vi "SentinelController v33.vi"() -> ()   [LabVIEW 2011] (continued)
                                n808 = local read "Number of data log entries hid"() -> (w3611:u32)
                                n809 = Unbundle(w3615) -> (w3614:i32)  [unwired: 3 out]
                                n810 = Unbundle(w3623) -> (w3621:u32)  [unwired: 1 out]
                                n811 = Unbundle(w3613) -> (w3612:i32)  [unwired: 3 out]
                                n812 = Unbundle(w3622) -> (w3620:u32)  [unwired: 1 out]
                                n813 = Number To Decimal String(number=w3629) -> (decimal integer string=w3638:string)  [unwired: 1 in]
                                n814 = Number To Decimal String(number=w3614) -> (decimal integer string=w3640:string)  [unwired: 1 in]
                                n815 = Number To Decimal String(number=w3630) -> (decimal integer string=w3642:string)  [unwired: 1 in]
                                n816 = Number To Decimal String(number=w3621) -> (decimal integer string=w3644:string)  [unwired: 1 in]
                                n817 = Number To Decimal String(number=w3631) -> (decimal integer string=w3647:string)  [unwired: 1 in]
                                n818 = Number To Decimal String(number=w3612) -> (decimal integer string=w3649:string)  [unwired: 1 in]
                                n819 = Number To Decimal String(number=w3632) -> (decimal integer string=w3651:string)  [unwired: 1 in]
                                n820 = Number To Decimal String(number=w3620) -> (decimal integer string=w3653:string)  [unwired: 1 in]
                                n821 = local read "Data log path and filename"() -> (w3619:path)
                                n822 = Get Date/Time String(want seconds? (F)=TRUE) -> (date string=w3627:string, time string=w3628:string)  [unwired: 2 in]
                                n823 = Number To Decimal String(number=w3611) -> (decimal integer string=w3616:string)  [unwired: 1 in]
                                n824 = Concatenate Strings(w3616, w3617, w3627, "   " ("string"), w3628, w3617, "H1 Alarming, H2 Nominal", w3617, w3636, w3617, "H1 Low Yield Alarm Limit: ", w3638, ", H1 yield = ", w3640, w3617, "H1 Low UPH Alarm Limit: ", w3642, ", H1 UPH = ", w3644, w3617, w3645, w3617, "H2 Low Yield Warning Limit: ", w3647, ", H2 yield = ", w3649, w3617, "H2 Low UPH Warning Limit: ", w3651, ", H2 UPH = ", w3653, w3617, w3617) -> (w3625:string)
                                n825 = call "SentinelDatalog.vi"("operation (0:open)"=T9."open", "String"=w3625, "data log path"=w3619) -> ()  [unwired: 8 in, 1 out]
                                }
                                frame "H1AH2W" {
                                w3664 = "\r\n"
                                n826 = local read "H1 online"() -> (w3681:bool)
                                n827 = local read "H2 online"() -> (w3682:bool)
                                n828 = local read "H2 UPH warning limit hid"() -> (w3679:dbl)
                                n829 = local read "H2  low yield warning"() -> (w3678:dbl)
                                n830 = local read "H1 UPH alarm limit hid"() -> (w3677:dbl)
                                n831 = local read "H1 low yield alarm"() -> (w3676:dbl)
                                n832 = local read "H1 UPH"() -> (w3670:cluster{u32, u32})
                                n833 = local read "H2 UPH"() -> (w3669:cluster{u32, u32})
                                n834 = local read "YieldMon"() -> (w3662:cluster{i32, i32, i32, i32})
                                n835 = local read "YieldMon"() -> (w3660:cluster{i32, i32, i32, i32})
                                n836 = case shown="True" w3681 {
                                tunnel: ["H1 Off-Line" "H1 On-Line"] -> w3683
                                frame False {
                                }
                                frame True {
                                }
                                }
                                n837 = case shown="True" w3682 {
                                tunnel: ["H2 Off-Line" "H2 On-Line"] -> w3692
                                frame False {
                                }
                                frame True {
                                }
                                }
                                n838 = local read "Number of data log entries hid"() -> (w3658:u32)
                                n839 = Unbundle(w3662) -> (w3661:i32)  [unwired: 3 out]
                                n840 = Unbundle(w3670) -> (w3668:u32)  [unwired: 1 out]
                                n841 = Unbundle(w3660) -> (w3659:i32)  [unwired: 3 out]
                                n842 = Unbundle(w3669) -> (w3667:u32)  [unwired: 1 out]
                                n843 = Number To Decimal String(number=w3676) -> (decimal integer string=w3685:string)  [unwired: 1 in]
                                n844 = Number To Decimal String(number=w3661) -> (decimal integer string=w3687:string)  [unwired: 1 in]
                                n845 = Number To Decimal String(number=w3677) -> (decimal integer string=w3689:string)  [unwired: 1 in]
                                n846 = Number To Decimal String(number=w3668) -> (decimal integer string=w3691:string)  [unwired: 1 in]
                                n847 = Number To Decimal String(number=w3678) -> (decimal integer string=w3694:string)  [unwired: 1 in]
                                n848 = Number To Decimal String(number=w3659) -> (decimal integer string=w3696:string)  [unwired: 1 in]
                                n849 = Number To Decimal String(number=w3679) -> (decimal integer string=w3698:string)  [unwired: 1 in]
                                n850 = Number To Decimal String(number=w3667) -> (decimal integer string=w3700:string)  [unwired: 1 in]
                                n851 = local read "Data log path and filename"() -> (w3666:path)
                                n852 = Get Date/Time String(want seconds? (F)=TRUE) -> (date string=w3674:string, time string=w3675:string)  [unwired: 2 in]
                                n853 = Number To Decimal String(number=w3658) -> (decimal integer string=w3663:string)  [unwired: 1 in]
                                n854 = Concatenate Strings(w3663, w3664, w3674, "   " ("string"), w3675, w3664, "H1 Alarming, H2 Warning", w3664, w3683, w3664, "H1 Low Yield Alarm Limit: ", w3685, ", H1 yield = ", w3687, w3664, "H1 Low UPH Alarm Limit: ", w3689, ", H1 UPH = ", w3691, w3664, w3692, w3664, "H2 Low Yield Warning Limit: ", w3694, ", H2 yield = ", w3696, w3664, "H2 Low UPH Warning Limit: ", w3698, ", H2 UPH = ", w3700, w3664) -> (w3672:string)
                                n855 = call "SentinelDatalog.vi"("operation (0:open)"=T9."open", "String"=w3672, "data log path"=w3666) -> ()  [unwired: 8 in, 1 out]
                                }
                                frame "H1AH2A" {
                                w3711 = "\r\n"
                                n856 = local read "H1 online"() -> (w3728:bool)
                                n857 = local read "H2 online"() -> (w3729:bool)
                                n858 = local read "H1 UPH alarm limit hid"() -> (w3724:dbl)
                                n859 = local read "H2 UPH alarm limit hid"() -> (w3726:dbl)
                                n860 = local read "H1 low yield alarm"() -> (w3723:dbl)
                                n861 = local read "H1 UPH"() -> (w3717:cluster{u32, u32})
                                n862 = local read "H2 low yield alarm"() -> (w3725:dbl)
                                n863 = local read "H2 UPH"() -> (w3716:cluster{u32, u32})
                                n864 = local read "YieldMon"() -> (w3709:cluster{i32, i32, i32, i32})
                                n865 = local read "YieldMon"() -> (w3708:cluster{i32, i32, i32, i32})
                                n866 = case shown="True" w3728 {
                                tunnel: ["H1 Off-Line" "H1 On-Line"] -> w3730
                                frame False {
                                }
                                frame True {
                                }
                                }
                                n867 = case shown="True" w3729 {
                                tunnel: ["H2 Off-Line" "H2 On-Line"] -> w3739
                                frame False {
                                }
                                frame True {
                                }
                                }
                                n868 = local read "Number of data log entries hid"() -> (w3705:u32)
                                n869 = Unbundle(w3709) -> (w3706:i32)  [unwired: 3 out]
                                n870 = Unbundle(w3717) -> (w3715:u32)  [unwired: 1 out]
                                n871 = Unbundle(w3708) -> (w3707:i32)  [unwired: 3 out]
                                n872 = Unbundle(w3716) -> (w3714:u32)  [unwired: 1 out]
                                n873 = Number To Decimal String(number=w3723) -> (decimal integer string=w3732:string)  [unwired: 1 in]
                                n874 = Number To Decimal String(number=w3706) -> (decimal integer string=w3734:string)  [unwired: 1 in]
                                n875 = Number To Decimal String(number=w3724) -> (decimal integer string=w3736:string)  [unwired: 1 in]
                                n876 = Number To Decimal String(number=w3715) -> (decimal integer string=w3738:string)  [unwired: 1 in]
                                n877 = Number To Decimal String(number=w3725) -> (decimal integer string=w3741:string)  [unwired: 1 in]
                                n878 = Number To Decimal String(number=w3707) -> (decimal integer string=w3743:string)  [unwired: 1 in]
                                n879 = Number To Decimal String(number=w3726) -> (decimal integer string=w3745:string)  [unwired: 1 in]
                                n880 = Number To Decimal String(number=w3714) -> (decimal integer string=w3747:string)  [unwired: 1 in]
                                n881 = local read "Data log path and filename"() -> (w3713:path)
                                n882 = Get Date/Time String(want seconds? (F)=TRUE) -> (date string=w3721:string, time string=w3722:string)  [unwired: 2 in]
                                n883 = Number To Decimal String(number=w3705) -> (decimal integer string=w3710:string)  [unwired: 1 in]
                                n884 = Concatenate Strings(w3710, w3711, w3721, "   " ("string"), w3722, w3711, "H1 Alarming, H2 Alarming", w3711, w3730, w3711, "H1 Low Yield Alarm Limit: ", w3732, ", H1 yield = ", w3734, w3711, "H1 Low UPH Alarm Limit: ", w3736, ", H1 UPH = ", w3738, w3711, w3739, w3711, "H2 Low Yield Alarm Limit: ", w3741, ", H2 yield = ", w3743, w3711, "H2 Low UPH Alarm Limit: ", w3745, ", H2 UPH = ", w3747, w3711, w3711) -> (w3719:string)
                                n885 = call "SentinelDatalog.vi"("operation (0:open)"=T9."open", "String"=w3719, "data log path"=w3713) -> ()  [unwired: 8 in, 1 out]
                                }
                                }
                                }
                                frame #2 {
                                n886 = Wait (ms)(milliseconds to wait=u32 100) -> ()  [unwired: 1 out]
                                }
                                frame #3 {
                                n887 = local read "Enable electronic notification of alarms"() -> (w3753:bool)
                                n888 = case shown="True" w3753 {
                                frame False {
                                }
                                frame True {
                                n889 = stacked-sequence {
                                frame #0 {
                                # "Email"
                                n890 = local read "Enable email notification"() -> (w3756:bool)
                                n891 = local read "Number of email alerts"() -> (w3755:u32)
                                n892 = Increment(x=w3755) -> (x+1=w3754:u32)
                                n893 = local write "Number of email alerts"(w3754) -> ()
                                n894 = case shown="True" w3756 {
                                frame False {
                                }
                                frame True {
                                n895 = flat-sequence {
                                tunnel: [w3763] -> w3758
                                tunnel: [w3771] -> w3757
                                tunnel: w3758 -> [w3771]
                                tunnel: w3757 -> [w3772]
                                frame #0 {
                                n896 = local read "Data log path and filename"() -> (w3768:path)
                                n897 = local read "Number of email alerts"() -> (w3762:u32)
                                n898 = Number To Decimal String(number=w3762) -> (decimal integer string=w3761:string)  [unwired: 1 in]
                                n899 = Strip Path(path=w3768) -> (stripped path=w3766:path, name=w3760:string)
                                n900 = Path To String(path=w3766) -> (string=w3765:string)
                                n901 = Concatenate Strings(w3765, "\\sent_#" ("string"), w3761, "_" ("string"), w3760) -> (w3769:string)
                                n902 = String To Path(string=w3769) -> (path=w3764:path)
                                n903 = Copy(10:w3764, 11:w3768) -> (3:w3763:path)  [unwired: 3 in, 2 out]
                                }
                                frame #1 {
                                n904 = Wait (ms)(milliseconds to wait=u32 1000) -> ()  [unwired: 1 out]
                                }
                                frame #2 {
                                n905 = local read "Email alert - engineer"() -> (w3774:string)
                                n906 = local read "Email alert - CC"() -> (w3773:string)
                                n907 = local read "Email alert - message"() -> (w3775:string)
                                n908 = call "email_alert.vi"("Email Alert - Message"=w3775, "Email Alert - Engineer"=w3774, "Email Alert - CC"=w3773, "Email ALert - Attachment"=w3772) -> ()  [unwired: 8 in]
                                }
                                }
                                }
                                }
                                }
                                frame #1 {
                                n909 = Wait (ms)(milliseconds to wait=u32 200) -> ()  [unwired: 1 out]
                                }
                                frame #2 {
                                # "text"
                                n910 = local read "Enable text notification"() -> (w3777:bool)
                                n911 = case shown="True" w3777 {
                                frame False {
                                }
                                frame True {
                                n912 = local read "Number of text alerts"() -> (w3781:u32)
                                n913 = Increment(x=w3781) -> (x+1=w3780:u32)
                                n914 = local write "Number of text alerts"(w3780) -> ()
                                n915 = local read "Number of email alerts"() -> (w3790:u32)
                                n916 = local read "Carrier"() -> (w3783:enum16{"T-Mobile", "AT&T", "Verizon", "Sprint"})
                                n917 = local read "Phone number"() -> (w3782:string)
                                n918 = local read "Body"() -> (w3779:string)
                                n919 = local read "Lot number"() -> (w3784:string)
                                n920 = local read "Subject"() -> (w3778:string)
                                n921 = Number To Decimal String(number=w3790) -> (decimal integer string=w3786:string)  [unwired: 1 in]
                                n922 = Concatenate Strings(w3779, ", # " ("string"), w3786, ", Lot Number: " ("string"), w3784) -> (w3791:string)
                                n923 = local write "Notifications Lot Display"(w3784) -> ()
                                n924 = call <userlib>:"Send SMS 2009.vi"("Body"=w3791, "Carrier"=w3783, "Subject"=w3778, "phone number"=w3782, "smtp server"="smtp.gmail.com", "password"="sentinelcontroller", "email username"="sentinelcontroller@gmail.com") -> ("Error Out"=w3789:errorcluster)  [unwired: 4 in]
                                n925 = Unbundle By Name(w3789) -> ("status"=w3788:bool)
                                n926 = case shown="True" w3788 {
                                frame False {
                                }
                                frame True {
                                n927 = One Button Dialog(message="Warning:\nError sending text message!\nTry changing the settings or\nswitch to email method", button name ("OK")="Dismiss") -> ()  [unwired: 1 out]
                                }
                                }
                                }
                                }
                                }
                                }
                                }
                                }
                                }
                                frame #4 {
                                n928 = Wait (ms)(milliseconds to wait=u32 100) -> ()  [unwired: 1 out]
                                }
                              }
                            }
                          }
                        }
                      }
                    }
                  }
                }
              }
              n929 = Wait (ms)(milliseconds to wait=u32 100) -> ()  [unwired: 1 out]
            }
            n930 = local read "Yield averaging"() -> (w350:u32)
            n931 = local read "UPH averaging"() -> (w349:u32)
            n932 = local read "Yield averaging"() -> (w351:u32)
            n933 = local read "UPH averaging"() -> (w352:u32)
            n934 = Initialize Array(w347, w350) -> (w348:i32[])
            n935 = Initialize Array(w346, w349) -> (w345:dbl[])
            n936 = Initialize Array(w354, w351) -> (w353:i32[])
            n937 = Initialize Array(w355, w352) -> (w356:dbl[])
            n938 = while {
              shift-right: [w3060] -> _
              shift-left: w346 -> [w3066]
              shift-right: [w3061] -> _
              shift-left: w345 -> [w3065]
              shift-right: [w3062] -> _
              shift-left: w347 -> [w3059]
              shift-right: [w3063] -> _
              shift-left: w348 -> [w3064]
              stop <- w3057 stop-if-true
              # "if there is now a lock, it is unlikely that the test time is going to be less than 100ms,\nso this is a relatively slow loop"
              n939 = local read "H2 Lock"() -> (w3056:bool)
              n940 = Wait (ms)(milliseconds to wait=u32 50) -> ()  [unwired: 1 out]
              n941 = case shown="True" w3056 {
                tunnel: w3066 -> [w3071 w3096]
                tunnel: w3065 -> [w3070 w3091]
                tunnel: w3064 -> [w3068 w3088]
                tunnel: [w3068 w3082] -> w3063
                tunnel: [w3069 w3080] -> w3062
                tunnel: [w3070 w3079] -> w3061
                tunnel: [w3071 w3078] -> w3060
                tunnel: w3059 -> [w3069 w3077]
                frame False {
                  n942 = local write "Calc H1 UPH"(u32 0 ("Sim H1 UPH")) -> ()
                }
                frame True {
                  n943 = flat-sequence {
                    tunnel: w3088 -> [w3099]
                    tunnel: w3077 -> [w3100]
                    tunnel: w3091 -> [w3101]
                    tunnel: w3096 -> [w3102]
                    tunnel: [w3102] -> w3087
                    tunnel: [w3101] -> w3086
                    tunnel: [w3100] -> w3085
                    tunnel: [w3099] -> w3084
                    tunnel: [w3115] -> w3095
                    tunnel: [w3114] -> w3092
                    tunnel: [w3113] -> w3090
                    tunnel: [w3112] -> w3089
                    tunnel: w3087 -> [w3115]
                    tunnel: w3086 -> [w3114]
                    tunnel: w3085 -> [w3113]
                    tunnel: w3084 -> [w3112]
                    tunnel: w3095 -> [w3141]
                    tunnel: [w3141] -> w3094
                    tunnel: [w3140] -> w3093
                    tunnel: w3092 -> [w3140]
                    tunnel: w3090 -> [w3130]
                    tunnel: w3089 -> [w3129]
                    tunnel: [w3128] -> w3083
                    tunnel: [w3127] -> w3081
                    tunnel: w3094 -> [w3167]
                    tunnel: w3093 -> [w3168]
                    tunnel: w3083 -> [w3186]
                    tunnel: w3081 -> [w3185]
                    tunnel: [w3186] -> w3076
                    tunnel: [w3185] -> w3075
                    tunnel: [w3164] -> w3074
                    tunnel: [w3163] -> w3073
                    tunnel: [w3201] -> w3078
                    tunnel: [w3202] -> w3079
                    tunnel: [w3203] -> w3080
                    tunnel: [w3204] -> w3082
                    tunnel: w3076 -> [w3204]
                    tunnel: w3075 -> [w3203]
                    tunnel: w3074 -> [w3202]
                    tunnel: w3073 -> [w3201]
                    frame #0 {
                      n944 = local read "H2 loop counter hid"() -> (w3097:u32)
                      n945 = Equal To 0?(x=w3097) -> (x = 0?=w3098:bool)
                      n946 = case shown="True" w3098 {
                        frame False {
                        }
                        frame True {
                          # "H2 first pass init"
                          n947 = local write "H2 Device Count"(0.0 ("H2 Device Count")) -> ()
                          n948 = local write "H2 measured  Index Time"(0.0 ("H2 Index Time")) -> ()
                          n949 = local write "H2 measured Test Time"(0.0 ("H2 Test Time")) -> ()
                          n950 = local write "H2 measured Wait Time"(0.0 ("H2 Wait Time")) -> ()
                          n951 = local read "H2 low UPH alarm (%)"() -> (w3106:dbl)
                          n952 = Divide(x=w3106, y=100.0) -> (x/y=w3105:dbl)
                          n953 = Bundle(0.0, w3105) -> (w3103:cluster{dbl, dbl})  [unwired: 1 in]
                          n954 = local write "H2 UPH"(w3103) -> ()
                        }
                      }
                    }
                    frame #1 {
                      # "H2 testing"
                      n955 = while {
                        stop <- w3119 stop-if-true
                        n956 = local read "H2 Lock"() -> (w3123:bool)
                        n957 = local read "POWER"() -> (w3118:bool)
                        n958 = local read "Run"() -> (w3116:bool)
                        n959 = Not(x=w3123) -> (.not. x?=w3117:bool)
                        n960 = Not(x=w3118) -> (.not. x?=w3121:bool)
                        n961 = Not(x=w3116) -> (.not. x?=w3120:bool)
                        n962 = Compound Arithmetic op=OR(w3117, w3121, w3120) -> (w3119:bool)
                        n963 = Wait (ms)(milliseconds to wait=u32 1) -> ()  [unwired: 1 out]
                      }
                    }
                    frame #2 {
                      n964 = local read "H2 cycle yield hid"() -> (w3124:dbl)
                      n965 = local read "H2 loop counter hid"() -> (w3125:u32)
                      n966 = local read "Yield averaging"() -> (w3126:u32)
                      n967 = local read "H2 low yield alarm"() -> (w3139:dbl)
                      n968 = local read "YieldMon"() -> (w3132:cluster{i32, i32, i32, i32})
                      n969 = local read "H2  low yield warning"() -> (w3138:dbl)
                      n970 = call "moving_avg_core.vi"("Array in"=w3129, "avg"=w3126, "accumulator in"=w3130, "i"=w3125, "data in"=w3124) -> ("Array out"=w3128:dbl[], "accumulator out"=w3127:dbl, "rolling avg out"=w3133:dbl)  [unwired: 4 in]
                      n971 = Unbundle(w3132) -> (w3131:i32)  [unwired: 3 out]
                      n972 = Less?(x=w3133, y=w3138) -> (x < y?=w3137:bool)
                      n973 = case shown="True" w3137 {
                        tunnel: w3133 -> [_ w3146]
                        tunnel: w3139 -> [_ w3145]
                        frame False {
                          n974 = local write "H2 nominal"(TRUE ("H1 nominal")) -> ()
                          n975 = local write "H2 warning"(FALSE ("H1 warning")) -> ()
                          n976 = local write "H2 alarm"(FALSE ("H1 warning")) -> ()
                        }
                        frame True {
                          n977 = Less?(x=w3146, y=w3145) -> (x < y?=w3147:bool)
                          n978 = case shown="True" w3147 {
                            frame False {
                              n979 = local write "H2 nominal"(FALSE ("H1 nominal")) -> ()
                              n980 = local write "H2 warning"(TRUE ("H1 warning")) -> ()
                              n981 = local write "H2 alarm"(FALSE ("H1 warning")) -> ()
                            }
                            frame True {
                              n982 = local read "H2 enable halt\non yield alarm"() -> (w3151:bool)
                              n983 = local write "H2 nominal"(FALSE ("H1 nominal")) -> ()
                              n984 = local write "H2 alarm"(TRUE ("H1 warning")) -> ()
                              n985 = local write "H2 warning"(FALSE ("H1 warning")) -> ()
                              n986 = case shown="True" w3151 {
                                frame False {
                                }
                                frame True {
                                n987 = local write "H2 online"(FALSE ("H1 Online")) -> ()
                                }
                              }
                            }
                          }
                        }
                      }
                      n988 = local read "H1 low yield alarm"() -> (w3136:dbl)
                      n989 = local read "H2 low yield alarm"() -> (w3135:dbl)
                      n990 = Bundle(w3131, "rolling avg out"=w3133, "H1 low yield alarm"=w3136, "H2 low yield alarm"=w3135) -> (w3134:T11)  [unwired: 1 in]
                      n991 = local write "YieldMon"(w3134) -> ()
                    }
                    frame #3 {
                      n992 = local read "H2 measured  Index Time"() -> (w3157:dbl)
                      n993 = local read "H2 measured Wait Time"() -> (w3156:dbl)
                      n994 = local read "H2 measured Test Time"() -> (w3158:dbl)
                      n995 = local read "H2 parallelism"() -> (w3170:u32)
                      n996 = local read "H2 lot yield mon"() -> (w3184:dbl)
                      n997 = local write "H2 IT (scycle)"(w3157) -> ()
                      n998 = local write "H2 TT (s/cycle)"(w3158) -> ()
                      n999 = local write "H2 WT (s/cycle)"(w3156) -> ()
                      n1000 = Compound Arithmetic op=ADD(w3157, w3158, w3156) -> (w3173:dbl)
                      n1001 = Compound Arithmetic op=ADD(w3157, w3158) -> (w3169:dbl)
                      n1002 = Multiply(x=w3170, y=3600.0 ("x")) -> (x*y=w3172:dbl)
                      n1003 = Divide(x=w3172, y=w3173) -> (x/y=w3183:dbl)
                      n1004 = Divide(x=w3184, y=w3169) -> (x/y=w3162:dbl)
                      n1005 = local write "H2 Single Handler UPH hid"(w3162) -> ()
                      n1006 = local read "H2 low UPH warning (%)"() -> (w3180:dbl)
                      n1007 = local read "H2 loop counter hid"() -> (w3166:u32)
                      n1008 = local read "Yield averaging"() -> (w3165:u32)
                      n1009 = local read "H2 low UPH alarm (%)"() -> (w3175:dbl)
                      n1010 = property on="H2 UPH" class="Knob (strict)"() -> ("Scale.Maximum"=w3181:dbl)  [unwired: 2 in, 2 out]
                      n1011 = Divide(x=w3180, y=100.0) -> (x/y=w3179:dbl)
                      n1012 = call "moving_avg_core.vi"("Array in"=w3168, "avg"=w3165, "accumulator in"=w3167, "i"=w3166, "data in"=w3183) -> ("Array out"=w3164:dbl[], "accumulator out"=w3163:dbl, "rolling avg out"=w3182:dbl)  [unwired: 4 in]
                      n1013 = Multiply(x=w3181, y=w3179) -> (x*y=w3161:dbl)
                      n1014 = Divide(x=w3175, y=100.0) -> (x/y=w3177:dbl)
                      n1015 = local write "H2 UPH warning limit hid"(w3161) -> ()
                      n1016 = Less?(x=w3182, y=w3161) -> (x < y?=w3174:bool)
                      n1017 = Multiply(x=w3181, y=w3177) -> (x*y=w3160:dbl)
                      n1018 = case shown="True" w3174 {
                        tunnel: w3182 -> [_ w3191]
                        tunnel: w3160 -> [_ w3190]
                        frame False {
                          n1019 = local write "H2 nominal 2"(TRUE ("H1 nominal")) -> ()
                          n1020 = local write "H2 warning 2"(FALSE ("H1 warning")) -> ()
                          n1021 = local write "H2 alarm 2"(FALSE ("H1 warning")) -> ()
                        }
                        frame True {
                          n1022 = Less?(x=w3191, y=w3190) -> (x < y?=w3192:bool)
                          n1023 = case shown="True" w3192 {
                            frame False {
                              n1024 = local write "H2 nominal 2"(FALSE ("H1 nominal")) -> ()
                              n1025 = local write "H2 warning 2"(TRUE ("H1 warning")) -> ()
                              n1026 = local write "H2 alarm 2"(FALSE ("H1 warning")) -> ()
                            }
                            frame True {
                              n1027 = local read "H2 enable halt\non UPH alarm"() -> (w3196:bool)
                              n1028 = local write "H2 alarm 2"(TRUE ("H1 warning")) -> ()
                              n1029 = local write "H2 warning 2"(FALSE ("H1 warning")) -> ()
                              n1030 = local write "H2 nominal 2"(FALSE ("H1 nominal")) -> ()
                              n1031 = case shown="True" w3196 {
                                frame False {
                                }
                                frame True {
                                n1032 = local write "H2 online"(FALSE ("H1 Online")) -> ()
                                }
                              }
                            }
                          }
                        }
                      }
                      n1033 = local write "H2 UPH alarm limit hid"(w3160) -> ()
                      n1034 = Bundle("rolling avg out"=w3182, w3160) -> (w3159:cluster{"rolling avg out":dbl, dbl})  [unwired: 1 in]
                      n1035 = local write "H2 UPH"(w3159) -> ()
                    }
                    frame #4 {
                      n1036 = while {
                        stop <- w3206 continue-if-true
                        n1037 = local read "H2 Lock"() -> (w3206:bool)
                        n1038 = Wait (ms)(milliseconds to wait=u32 10) -> ()  [unwired: 1 out]
                      }
                    }
                  }
                }
              }
              n1039 = local read "POWER"() -> (w3058:bool)
              n1040 = Not(x=w3058) -> (.not. x?=w3057:bool)
            }
            n1041 = while {
              shift-right: [w3937] -> _
              shift-left: w355 -> [w3940]
              shift-right: [w3938] -> _
              shift-left: w356 -> [w3939]
              shift-right: [w3933] -> _
              shift-left: w354 -> [w3936]
              shift-right: [w3934] -> _
              shift-left: w353 -> [w3935]
              stop <- w3932 stop-if-true
              # "if there is now a lock, it is unlikely that the test time is going to be less than 100ms,\nso this is a relatively slow loop"
              n1042 = local read "H1 Lock"() -> (w3931:bool)
              n1043 = case shown="True" w3931 {
                tunnel: w3940 -> [w3946 w3971]
                tunnel: w3939 -> [w3945 w3966]
                tunnel: [w3945 w3965] -> w3938
                tunnel: [w3946 w3964] -> w3937
                tunnel: w3936 -> [w3944 w3962]
                tunnel: w3935 -> [w3943 w3960]
                tunnel: [w3943 w3958] -> w3934
                tunnel: [w3944 w3956] -> w3933
                frame False {
                  n1044 = local write "Calc H1 UPH"(u32 0 ("Sim H1 UPH")) -> ()
                }
                frame True {
                  n1045 = flat-sequence {
                    tunnel: w3960 -> [w3974]
                    tunnel: w3962 -> [w3975]
                    tunnel: w3966 -> [w3976]
                    tunnel: w3971 -> [w3977]
                    tunnel: [w3977] -> w3955
                    tunnel: [w3976] -> w3954
                    tunnel: [w3975] -> w3953
                    tunnel: [w3974] -> w3952
                    tunnel: [w3990] -> w3970
                    tunnel: [w3989] -> w3967
                    tunnel: [w3988] -> w3963
                    tunnel: [w3987] -> w3961
                    tunnel: w3955 -> [w3990]
                    tunnel: w3954 -> [w3989]
                    tunnel: w3953 -> [w3988]
                    tunnel: w3952 -> [w3987]
                    tunnel: w3970 -> [w4005]
                    tunnel: [w4005] -> w3969
                    tunnel: [w4004] -> w3968
                    tunnel: w3967 -> [w4004]
                    tunnel: w3963 -> [w4003]
                    tunnel: w3961 -> [w4002]
                    tunnel: [w4001] -> w3959
                    tunnel: [w4000] -> w3957
                    tunnel: w3969 -> [w4043]
                    tunnel: w3968 -> [w4042]
                    tunnel: w3959 -> [w4039]
                    tunnel: w3957 -> [w4038]
                    tunnel: [w4041] -> w3951
                    tunnel: [w4040] -> w3950
                    tunnel: [w4039] -> w3949
                    tunnel: [w4038] -> w3948
                    tunnel: [w4078] -> w3956
                    tunnel: [w4079] -> w3958
                    tunnel: [w4080] -> w3964
                    tunnel: [w4081] -> w3965
                    tunnel: w3951 -> [w4081]
                    tunnel: w3950 -> [w4080]
                    tunnel: w3949 -> [w4079]
                    tunnel: w3948 -> [w4078]
                    frame #0 {
                      n1046 = local read "H1 loop counter hid"() -> (w3973:u32)
                      n1047 = Equal To 0?(x=w3973) -> (x = 0?=w3972:bool)
                      n1048 = case shown="True" w3972 {
                        frame False {
                        }
                        frame True {
                          n1049 = local read "H1 low UPH alarm (%)"() -> (w3982:dbl)
                          n1050 = local write "H1 measured Index Time"(0.0 ("H1 Index Time")) -> ()
                          n1051 = local write "H1 measured Wait Time"(0.0 ("H1 Wait Time")) -> ()
                          n1052 = local write "H1 Device Count"(0.0 ("H1 Device Count")) -> ()
                          n1053 = local write "H1 measured Test Time"(0.0 ("H1 Test Time")) -> ()
                          n1054 = Divide(x=w3982, y=100.0) -> (x/y=w3980:dbl)
                          n1055 = Bundle("y"=0.0, w3980) -> (w3978:cluster{"y":dbl, dbl})  [unwired: 1 in]
                          n1056 = local write "H1 UPH"(w3978) -> ()
                        }
                      }
                    }
                    frame #1 {
                      # "H1 testing"
                      n1057 = while {
                        stop <- w3994 stop-if-true
                        n1058 = local read "H1 Lock"() -> (w3998:bool)
                        n1059 = local read "POWER"() -> (w3992:bool)
                        n1060 = local read "Run"() -> (w3991:bool)
                        n1061 = Wait (ms)(milliseconds to wait=u32 1) -> ()  [unwired: 1 out]
                        n1062 = Not(x=w3998) -> (.not. x?=w3993:bool)
                        n1063 = Not(x=w3992) -> (.not. x?=w3996:bool)
                        n1064 = Not(x=w3991) -> (.not. x?=w3995:bool)
                        n1065 = Compound Arithmetic op=OR(w3993, w3996, w3995) -> (w3994:bool)
                      }
                    }
                    frame #2 {
                      n1066 = local read "H1 cycle yield hid"() -> (w4008:dbl)
                      n1067 = local read "H1 loop counter hid"() -> (w4007:u32)
                      n1068 = local read "Yield averaging"() -> (w4006:u32)
                      n1069 = local read "H1 low yield warning"() -> (w4016:dbl)
                      n1070 = local read "H1 low yield alarm"() -> (w4014:dbl)
                      n1071 = call "moving_avg_core.vi"("Array in"=w4002, "avg"=w4006, "accumulator in"=w4003, "i"=w4007, "data in"=w4008) -> ("Array out"=w4001:dbl[], "accumulator out"=w4000:dbl, "rolling avg out"=w4011:dbl)  [unwired: 4 in]
                      n1072 = Less?(x=w4011, y=w4016) -> (x < y?=w4015:bool)
                      n1073 = case shown="True" w4015 {
                        tunnel: w4011 -> [_ w4022]
                        tunnel: w4014 -> [_ w4021]
                        frame False {
                          n1074 = local write "H1 alarm"(FALSE ("H1 warning")) -> ()
                          n1075 = local write "H1 warning"(FALSE ("H1 warning")) -> ()
                          n1076 = local write "H1 nominal"(TRUE ("H1 nominal")) -> ()
                        }
                        frame True {
                          n1077 = Less?(x=w4022, y=w4021) -> (x < y?=w4020:bool)
                          n1078 = case shown="True" w4020 {
                            frame False {
                              n1079 = local write "H1 alarm"(FALSE ("H1 warning")) -> ()
                              n1080 = local write "H1 warning"(TRUE ("H1 warning")) -> ()
                              n1081 = local write "H1 nominal"(FALSE ("H1 nominal")) -> ()
                            }
                            frame True {
                              n1082 = local read "H1 enable halt\non yield alarm"() -> (w4026:bool)
                              n1083 = local write "H1 nominal"(FALSE ("H1 nominal")) -> ()
                              n1084 = local write "H1 warning"(FALSE ("H1 warning")) -> ()
                              n1085 = local write "H1 alarm"(TRUE ("H1 warning")) -> ()
                              n1086 = case shown="True" w4026 {
                                frame False {
                                }
                                frame True {
                                n1087 = local write "H1 online"(FALSE ("H1 Online")) -> ()
                                }
                              }
                            }
                          }
                        }
                      }
                      n1088 = local read "YieldMon"() -> (w4010:cluster{i32, i32, i32, i32})
                      n1089 = local read "H1 low yield alarm"() -> (w4013:dbl)
                      n1090 = local read "H2 low yield alarm"() -> (w4012:dbl)
                      n1091 = Unbundle(w4010) -> (w3999:i32)  [unwired: 3 out]
                      n1092 = Bundle("rolling avg out"=w4011, w3999, "H1 low yield alarm"=w4013, "H2 low yield alarm"=w4012) -> (w4009:T12)  [unwired: 1 in]
                      n1093 = local write "YieldMon"(w4009) -> ()
                    }
                    frame #3 {
                      n1094 = local read "H1 measured Index Time"() -> (w4033:dbl)
                      n1095 = local read "H1 measured Wait Time"() -> (w4031:dbl)
                      n1096 = local read "H1 measured Test Time"() -> (w4032:dbl)
                      n1097 = local read "H1 parallelism"() -> (w4050:u32)
                      n1098 = local read "H1 loop counter hid"() -> (w4045:u32)
                      n1099 = local read "UPH averaging"() -> (w4044:u32)
                      n1100 = local read "H1 low UPH warning (%)"() -> (w4054:dbl)
                      n1101 = local write "H1 IT (s/cycle)"(w4033) -> ()
                      n1102 = local write "H1 TT (s/cycle)"(w4032) -> ()
                      n1103 = local write "H1 WT (s/cycle)"(w4031) -> ()
                      n1104 = Compound Arithmetic op=ADD(w4033, w4032, w4031) -> (w4046:dbl)
                      n1105 = Compound Arithmetic op=ADD(w4033, w4032) -> (w4053:dbl)
                      n1106 = Multiply(x=w4050, y=u32 3600 ("x")) -> (x*y=w4052:u32)
                      n1107 = Divide(x=w4052, y=w4053) -> (x/y=w4036:dbl)
                      n1108 = local read "H1 low UPH alarm (%)"() -> (w4059:dbl)
                      n1109 = local write "H1 Single Handler UPH hid"(w4036) -> ()
                      n1110 = property on="H1 UPH" class="Knob (strict)"() -> ("Scale.Maximum"=w4061:dbl)  [unwired: 2 in, 2 out]
                      n1111 = Divide(x=w4054, y=100.0) -> (x/y=w4055:dbl)
                      n1112 = Multiply(x=w4061, y=w4055) -> (x*y=w4034:dbl)
                      n1113 = Divide(x=w4059, y=100.0) -> (x/y=w4057:dbl)
                      n1114 = local write "H1 UPH warning limit hid"(w4034) -> ()
                      n1115 = Multiply(x=w4061, y=w4057) -> (x*y=w4035:dbl)
                      n1116 = local write "H1 UPH alarm limit hid"(w4035) -> ()
                      n1117 = local read "H1 parallelism"() -> (w4049:u32)
                      n1118 = Multiply(x=w4049, y=u32 3600 ("x")) -> (x*y=w4047:u32)
                      n1119 = Divide(x=w4047, y=w4046) -> (x/y=w4063:dbl)
                      n1120 = call "moving_avg_core.vi"("Array in"=w4042, "avg"=w4044, "accumulator in"=w4043, "i"=w4045, "data in"=w4063) -> ("Array out"=w4041:dbl[], "accumulator out"=w4040:dbl, "rolling avg out"=w4062:dbl)  [unwired: 4 in]
                      n1121 = Less?(x=w4062, y=w4034) -> (x < y?=w4060:bool)
                      n1122 = case shown="True" w4060 {
                        tunnel: w4062 -> [_ w4068]
                        tunnel: w4035 -> [_ w4067]
                        frame False {
                          n1123 = local write "H1 alarm 2"(FALSE ("H1 warning")) -> ()
                          n1124 = local write "H1 nominal 2"(TRUE ("H1 nominal")) -> ()
                          n1125 = local write "H1 warning 2"(FALSE ("H1 warning")) -> ()
                        }
                        frame True {
                          n1126 = Less?(x=w4068, y=w4067) -> (x < y?=w4069:bool)
                          n1127 = case shown="True" w4069 {
                            frame False {
                              n1128 = local write "H1 nominal 2"(FALSE ("H1 nominal")) -> ()
                              n1129 = local write "H1 warning 2"(TRUE ("H1 warning")) -> ()
                              n1130 = local write "H1 alarm 2"(FALSE ("H1 warning")) -> ()
                            }
                            frame True {
                              n1131 = local read "H1 enable halt\non UPH alarm"() -> (w4073:bool)
                              n1132 = local write "H1 warning 2"(FALSE ("H1 warning")) -> ()
                              n1133 = local write "H1 alarm 2"(TRUE ("H1 warning")) -> ()
                              n1134 = local write "H1 nominal 2"(FALSE ("H1 nominal")) -> ()
                              n1135 = case shown="True" w4073 {
                                frame False {
                                }
                                frame True {
                                n1136 = local write "H1 online"(FALSE ("H1 Online")) -> ()
                                }
                              }
                            }
                          }
                        }
                      }
                      n1137 = Bundle("rolling avg out"=w4062, w4035) -> (w4037:cluster{"rolling avg out":dbl, dbl})  [unwired: 1 in]
                      n1138 = local write "H1 UPH"(w4037) -> ()
                    }
                    frame #4 {
                      n1139 = while {
                        stop <- w4083 continue-if-true
                        n1140 = local read "H1 Lock"() -> (w4083:bool)
                        n1141 = Wait (ms)(milliseconds to wait=u32 10) -> ()  [unwired: 1 out]
                      }
                    }
                  }
                }
              }
              n1142 = Wait (ms)(milliseconds to wait=u32 50) -> ()  [unwired: 1 out]
              n1143 = local read "POWER"() -> (w3942:bool)
              n1144 = Not(x=w3942) -> (.not. x?=w3932:bool)
            }
            n1145 = while {
              stop <- w1236 continue-if-true
              n1146 = while {
                stop <- w1238 stop-if-true
                n1147 = event shown="[1] \"H1 online\": Value Change" {
                  selector: _ -> [_ _]
                  dyn-events: _ -> [_ _]
                  timeout: -1 -> [_ _]
                  tunnel: [_ TRUE] -> w1238
                  event Timeout {
                    n1148 = event-data() -> ()  [unwired: 1 in, 2 out]
                  }
                  event "H1 online": Value Change {
                    n1149 = event-data() -> ()  [unwired: 1 in, 5 out]
                    n1150 = local read "Enable data logging of all events"() -> (w1239:bool)
                    n1151 = case shown="True" w1239 {
                      frame False {
                      }
                      frame True {
                        w1243 = "\r\n"
                        n1152 = Get Date/Time String(want seconds? (F)=TRUE) -> (date string=w1248:string, time string=w1247:string)  [unwired: 2 in]
                        n1153 = local read "H1 online"() -> (w1245:bool)
                        n1154 = case shown="False" w1245 {
                          tunnel: ["H1 Off-Line" "H1 On-Line"] -> w1244
                          frame False {
                          }
                          frame True {
                          }
                        }
                        n1155 = local read "Data log path and filename"() -> (w1242:path)
                        n1156 = Concatenate Strings(w1248, "   " ("string"), w1247, w1243, "Change in H1 Status: ", w1244, w1243, w1243) -> (w1250:string)
                        n1157 = call "SentinelDatalog.vi"("operation (0:open)"=T9."open", "String"=w1250, "data log path"=w1242) -> ()  [unwired: 8 in, 1 out]
                      }
                    }
                  }
                }
              }
              n1158 = local read "POWER"() -> (w1236:bool)
            }
            n1159 = while {
              stop <- w1218 continue-if-true
              n1160 = while {
                stop <- w1220 stop-if-true
                n1161 = event shown="[1] \"H2 online\": Value Change" {
                  selector: _ -> [_ _]
                  dyn-events: _ -> [_ _]
                  timeout: -1 -> [_ _]
                  tunnel: [_ TRUE] -> w1220
                  event Timeout {
                    n1162 = event-data() -> ()  [unwired: 1 in, 2 out]
                  }
                  event "H2 online": Value Change {
                    n1163 = event-data() -> ()  [unwired: 1 in, 5 out]
                    n1164 = local read "Enable data logging of all events"() -> (w1221:bool)
                    n1165 = case shown="True" w1221 {
                      frame False {
                      }
                      frame True {
                        w1225 = "\r\n"
                        n1166 = local read "H2 online"() -> (w1227:bool)
                        n1167 = case shown="False" w1227 {
                          tunnel: ["H2 Off-Line" "H2 On-Line"] -> w1226
                          frame False {
                          }
                          frame True {
                          }
                        }
                        n1168 = local read "Data log path and filename"() -> (w1224:path)
                        n1169 = Get Date/Time String(want seconds? (F)=TRUE) -> (date string=w1230:string, time string=w1229:string)  [unwired: 2 in]
                        n1170 = Concatenate Strings(w1230, "   " ("string"), w1229, w1225, "Change in H2 Status: ", w1226, w1225, w1225) -> (w1232:string)
                        n1171 = call "SentinelDatalog.vi"("operation (0:open)"=T9."open", "String"=w1232, "data log path"=w1224) -> ()  [unwired: 8 in, 1 out]
                      }
                    }
                  }
                }
              }
              n1172 = local read "POWER"() -> (w1218:bool)
            }
            n1173 = while {
              stop <- w1366 continue-if-true
              n1174 = local read "Tester online"() -> (w1367:bool)
              n1175 = case shown="True" w1367 {
                frame False {
                }
                frame True {
                  n1176 = flat-sequence {
                    frame #0 {
                      n1177 = local write "Exit SC handler StMach hid"(FALSE ("Exit tester state machine hid")) -> ()
                      n1178 = local write "SC handler states hid"(SC_handler_states."initializing bus" ("SC virtual handler states")) -> ()
                    }
                    frame #1 {
                      n1179 = flat-sequence {
                        tunnel: [w1374] -> w1371
                        tunnel: [w1373] -> w1372
                        frame #0 {
                          w1373 = 0.0
                          # "These are consumed in the \"responding to sites\"\nstate when at least one handler has sites ready.  \nIt is executed only after one cycle. At that point,\nthere is at least one test period and one wait period\nto make a utilization calculation."
                          n1180 = local read "Utilization averaging"() -> (w1375:i32)
                          n1181 = Initialize Array(w1373, w1375) -> (w1374:dbl[])
                        }
                      }
                      n1182 = while {
                        shift-right: [w1383] -> _
                        shift-left: w1372 -> [w1378]
                        shift-right: [w1379] -> _
                        shift-left: w1371 -> [w1377]
                        i -> [w1376]
                        stop <- w1380 stop-if-true
                        n1183 = flat-sequence {
                          tunnel: [w1389] -> w1382
                          tunnel: [w1388] -> w1381
                          tunnel: w1378 -> [w1387]
                          tunnel: w1377 -> [w1386]
                          tunnel: [w2194] -> w1379
                          tunnel: [w2195] -> w1383
                          tunnel: w1382 -> [w2195]
                          tunnel: w1381 -> [w2194]
                          frame #0 {
                            n1184 = local read "SC handler states hid"() -> (w1385:T6)
                            n1185 = case shown="\"waiting on serial poll\"" w1385 {
                              tunnel: w1387 -> [w1390 w1411 w1438 w1471 w1545 w1561 w1568 w1601 w1633 w1655 w1692 w1805 w1923 w1934 w2036 w2061 w2074 w2175 w2186]
                              tunnel: [w1391 w1412 w1439 w1472 w1546 w1560 w1569 w1600 w1632 w1654 w1689 w1802 w1924 w1933 w2035 w2060 w2073 w2174 w2185] -> w1388
                              tunnel: w1386 -> [w1391 w1412 w1439 w1472 w1546 w1560 w1569 w1600 w1632 w1654 w1691 w1804 w1924 w1933 w2035 w2060 w2073 w2174 w2185]
                              tunnel: [w1390 w1411 w1438 w1471 w1545 w1561 w1568 w1601 w1633 w1655 w1690 w1803 w1923 w1934 w2036 w2061 w2074 w2175 w2186] -> w1389
                              frame "initializing bus", Default {
                                n1186 = flat-sequence {
                                frame #0 {
                                n1187 = local write "VISA bus 0 close error"(FALSE ("VISA bus 0 close error")) -> ()
                                }
                                frame #1 {
                                w1400 = T13 1073684500 items=["Service Request"=1073684491, "Trigger"=3221168138, "Clear"=1073684493, "VXI Signal"=1073684512, "VXI/VME Interrupt"=3221168161, "VXI/VME Sysfail"=1073684509, "VXI/VME Sysreset"=1073684510, "GPIB CIC"=1073684498, "GPIB Talk"=1073684499, "GPIB Listen"=1073684500, "PXI Interrupt"=1073684514, "Serial Break"=1073684515, "Serial TermChar"=1073684516, "Serial CTS"=1073684521, "Serial DSR"=1073684522, "Serial DCD"=1073684524, "Serial RI"=1073684526, "Serial Character"=1073684533, "USB Interrupt"=1073684535, "All Enabled"=1073709055] ("Event Type")
                                n1188 = local read "SentCtrl listens to tester at"() -> (w1397:refnum<visa-resource-name>)
                                n1189 = local read "GPIB wait timeout hid"() -> (w1395:u32)
                                n1190 = VISA Open(VISA resource name=w1397) -> (VISA resource name=w1402:refnum<visa-resource-name>, error out=w1401:errorcluster)  [unwired: 1 in, 3 out]
                                n1191 = Unbundle By Name(w1401) -> ()  [unwired: 1 out]
                                n1192 = property class="GPIB BoardInterface"(reference=w1402, error in=w1401, "General Settings:Timeout Value"=w1395) -> (reference out=w1399:refnum<visa-resource-name>, error out=w1398:errorcluster)
                                n1193 = VISA Enable Event(8:w1398, 10:w1400, 11:w1399) -> (0:w1394:errorcluster, 3:→"VISA bus 0 resource name out hid":refnum<visa-resource-name>)  [unwired: 1 out]
                                "VISA bus 0 error out hid" <- w1394
                                n1194 = Unbundle By Name(w1394) -> ("status"=w1393:bool)
                                n1195 = local write "VISA bus 0 open error"(w1393) -> ()
                                }
                                frame #2 {
                                n1196 = Concatenate Strings("Bus 0 initializing " ("string"), "\r\n") -> (w1404:string)
                                n1197 = local write "GPIB Bus 0 traffic"(w1404) -> ()
                                }
                                frame #3 {
                                n1198 = local write "Exit SC handler StMach hid"(FALSE ("Exit tester state machine hid")) -> ()
                                }
                                frame #4 {
                                n1199 = local read "Tester Handler Config"() -> (w1407:T2)
                                n1200 = case shown="\"Seiko-Epson NS6040\"" w1407 {
                                frame "Multitest", Default {
                                n1201 = local write "SC handler states hid"(SC_handler_states."waiting on event" ("SC Test Interface States")) -> ()
                                }
                                frame "DeltaDesign" {
                                n1202 = local write "SC handler states hid"(SC_handler_states."waiting on event" ("SC Test Interface States")) -> ()
                                }
                                frame "Seiko-Epson NS6040" {
                                n1203 = local write "SC handler states hid"(SC_handler_states."waiting on serial poll" ("SC Test Interface States")) -> ()
                                }
                                }
                                }
                                }
                              }
                              frame "waiting on event" {
                                n1204 = flat-sequence {
                                frame #0 {
                                n1205 = local read "GPIB Bus 0 traffic"() -> (w1413:string)
                                n1206 = Concatenate Strings(w1413, "\r\n", "Bus 0 waiting on event" ("string")) -> (w1416:string)
                                n1207 = local write "GPIB Bus 0 traffic"(w1416) -> ()
                                }
                                frame #1 {
                                n1208 = local read "VISA bus 0 resource name out hid"() -> (w1426:refnum<visa-resource-name>)
                                n1209 = local read "VISA bus 0 error out hid"() -> (w1425:errorcluster)
                                n1210 = local read "GPIB wait timeout hid"() -> (w1424:u32)
                                n1211 = VISA Wait on Event(7:w1424, 8:w1425, 11:w1426) -> (0:w1417:errorcluster, 3:w1418:refnum<visa-resource-name>)  [unwired: 2 in, 2 out]
                                n1212 = local write "VISA bus 0 resource name out hid"(w1418) -> ()
                                n1213 = local write "VISA bus 0 error out hid"(w1417) -> ()
                                n1214 = Unbundle By Name(w1417) -> ("status"=w1421:bool)
                                n1215 = Unbundle By Name(w1417) -> ("code"=w1423:i32)
                                n1216 = Equal?(x=w1423, y=-1073807339) -> (x = y?=w1420:bool)
                                n1217 = Or(x=w1421, y=w1420) -> (x .or. y?=w1419:bool)
                                n1218 = case shown="False" w1419 {
                                tunnel: w1418 -> [_ w1429]
                                tunnel: w1417 -> [_ w1428]
                                frame False {
                                n1219 = local write "SC handler states hid"(SC_handler_states."reading" ("SC Test Interface States")) -> ()
                                }
                                frame True {
                                n1220 = flat-sequence {
                                tunnel: w1429 -> [w1433]
                                tunnel: w1428 -> [w1432]
                                frame #0 {
                                n1221 = VISA Close(VISA resource name=w1433, error in (no error)=w1432) -> (error out=w1431:errorcluster)
                                n1222 = Unbundle By Name(w1431) -> ("status"=w1430:bool)
                                n1223 = local write "VISA bus 0 close error"(w1430) -> ()
                                }
                                frame #1 {
                                n1224 = Concatenate Strings("GPIB bus 0 error or time out waiting on event,\nclosing Bus 0 and re-initializing." ("string"), "\r\n") -> (w1436:string)
                                n1225 = local write "GPIB Bus 0 traffic"(w1436) -> ()
                                }
                                frame #2 {
                                n1226 = local write "SC handler states hid"(SC_handler_states."initializing bus" ("SC Test Interface States")) -> ()
                                }
                                }
                                }
                                }
                                }
                                }
                              }
                              frame "waiting on serial poll" {
                                n1227 = flat-sequence {
                                frame #0 {
                                n1228 = local read "H1 Ready with sites"() -> (w1442:bool)
                                n1229 = local read "H2 Ready with sites"() -> (w1441:bool)
                                n1230 = Or(x=w1442, y=w1441) -> (x .or. y?=w1440:bool)
                                n1231 = case shown="True" w1440 {
                                frame False {
                                n1232 = property class="GPIB BoardInterface"(reference=refnum<visa-resource-name> "GPIB0::INTFC", "Device STB"=u8 0 ("Message Based Settings:Device Status Byte")) -> ()  [unwired: 1 in, 2 out]
                                }
                                frame True {
                                n1233 = property class="GPIB BoardInterface"(reference=refnum<visa-resource-name> "GPIB0::INTFC", "Device STB"=u8 65 ("Message Based Settings:Device Status Byte")) -> ()  [unwired: 1 in, 2 out]
                                }
                                }
                                }
                                frame #1 {
                                n1234 = local read "GPIB Bus 0 traffic"() -> (w1447:string)
                                n1235 = Concatenate Strings(w1447, "\r\n", "Bus 0 waiting on SPOLL" ("string")) -> (w1450:string)
                                n1236 = local write "GPIB Bus 0 traffic"(w1450) -> ()
                                }
                                frame #2 {
                                w1463 = "1"
                                w1453 = "%08b"  # format string
                                # "If the status bytes was x1xx xxx1 and now it is x0xx xxx0, then a serial poll ocurred, otherwise, it was a simple write event from the tester the BUS0"
                                n1237 = property class="GPIB BoardInterface"(reference=refnum<visa-resource-name> "GPIB0::INTFC") -> ("Device STB"=w1464:u8)  [unwired: 1 in, 2 out]
                                n1238 = Format Into String "Format Into String"(format string=w1453, w1464) -> (resulting string=w1462:string)  [unwired: 2 in, 1 out]
                                n1239 = String Subset(string=w1462, offset (0)=1, length (rest)=1 ("length (rest)")) -> (substring=w1457:string)
                                n1240 = String Subset(string=w1462, offset (0)=7, length (rest)=1 ("length (rest)")) -> (substring=w1456:string)
                                n1241 = Equal?(x=w1457, y=w1463) -> (x = y?=w1458:bool)
                                n1242 = Equal?(x=w1463, y=w1456) -> (x = y?=w1459:bool)
                                n1243 = And(x=w1458, y=w1459) -> (x .and. y?=w1451:bool)
                                n1244 = case shown="False" w1451 {
                                frame False {
                                n1245 = local write "SC handler states hid"(SC_handler_states."waiting on serial poll" ("SC Test Interface States")) -> ()
                                n1246 = Wait (ms)(milliseconds to wait=u32 5) -> ()  [unwired: 1 out]
                                }
                                frame True {
